vi "Configure Sequence Reset.vi"(0 "VISA resource name":refnum<visa-resource-name>, 1 "Reset (0: No Reset)":u16(ring) items=["No Reset", "Pattern 1 Entered", "Pattern 1 Exited", "Edge 1", "Pattern 1 and Edge 1", "Pattern 2 Entered", "Pattern 2 Exited", "Edge 2", "Timeout"], 11 "error in (no error)":errorcluster, 12 "Timeout (100.0E-9)":dbl=1e-07 format="%^#_6g") -> (4 "VISA resource name out":refnum<visa-resource-name>, 15 "error out":errorcluster)   [LabVIEW 2017, in "Agilent 6000 Series.lvlib"]
doc: "This VI configures the Sequence trigger. You specify the reset and timeout with the Reset and Timeout parameters.\n\n<B>NOTE:</B>\n\nThis VI is only valid for 6000 Series models. An error will be thrown if this VI is run with 5000 Series scopes."
uses:
  <instrlib>/Agilent 6000 Series/Agilent 6000 Series.lvlib
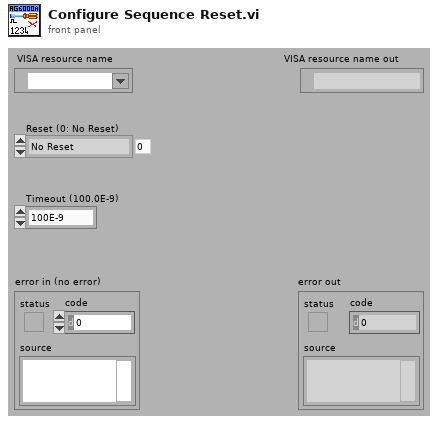
[diagram p1: front panel]
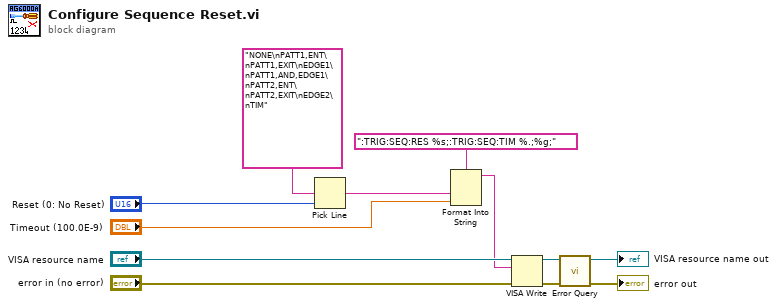
[diagram p0: block diagram]
diagram:
  n1 = Pick Line(multi-line string="NONE\nPATT1,ENT\nPATT1,EXIT\nEDGE1\nPATT1,AND,EDGE1\nPATT2,ENT\nPATT2,EXIT\nEDGE2\nTIM", line index="Reset (0: No Reset)") -> (output string=w2:string)  [unwired: 1 in]
  n2 = Format Into String(format string=":TRIG:SEQ:RES %s;:TRIG:SEQ:TIM %.;%g;" ("Source Command"), w2, "Timeout (100.0E-9)") -> (resulting string=w5:string)  [unwired: 2 in, 1 out]
  n3 = VISA Write(VISA resource name="VISA resource name", write buffer=w5, error in (no error)="error in (no error)") -> (VISA resource name out=w8:refnum<visa-resource-name>, error out=w7:errorcluster)  [unwired: 1 out]
  n4 = call <instrlib>:"Error Query.vi"("error in (no error)"=w7, "VISA resource name"=w8) -> ("error out"=→"error out":errorcluster, "VISA resource name out"=→"VISA resource name out":refnum<visa-resource-name>)  [unwired: 6 in, 2 out]
